vi "DAQ.Create Sample Clock.vi"(8 "error in (no error)":errorcluster, 11 "Instrument.DAQ":refnum<class "Instrument.DAQ.lvclass">) -> (0 "error out":errorcluster, 3 "Instrument.DAQ":refnum<class "Instrument.DAQ.lvclass">)   [LabVIEW 2019, in "Instrument.Lockin.lvlib" / "Instrument.DAQ.lvclass"]
uses:
  Instrument.DAQ.lvclass
  Instrument.DAQ.lvclass/Instrument.DAQ.ctl
  <vilib>/DAQmx/configure/timing.llb/DAQmx Timing (Sample Clock).vi
  <resource>/objmgr/daqmx.rc
panel:
  out "Fs (S/s) 3":dbl[](array[numeric]) format="%#_13g"
  out "Fs (S/s) 2":dbl[](array[numeric]) format="%#_13g"
  out "Output.Onboard Buffer":u32[](array[numeric])
  out "Output.Buffer":u32[](array[numeric])
  out "Input.Onboard Buffer":u32[](array[numeric])
  out "Input.Buffer":u32[](array[numeric])
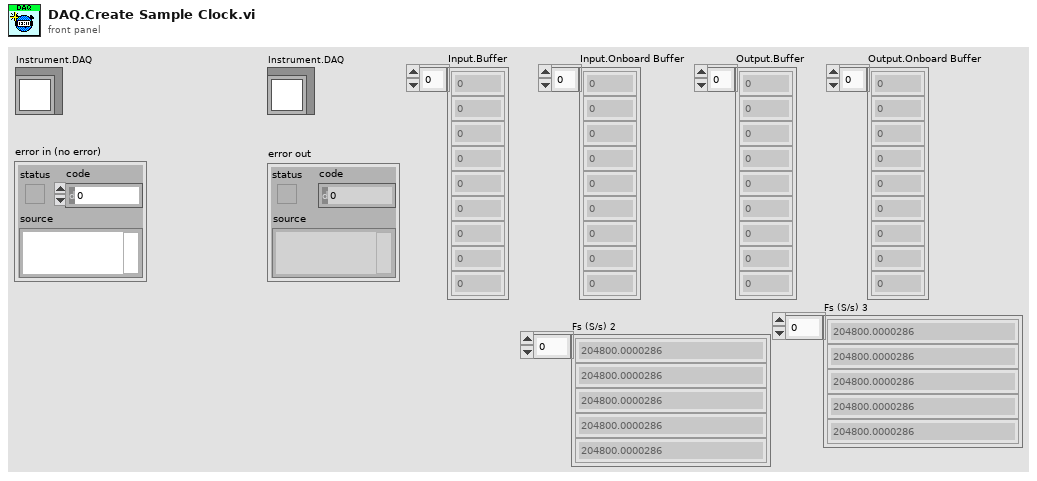
[diagram p1: front panel]
types:
  T1 = typedef "Instrument.Lockin.lvlib/Instrument.DAQ.lvclass/DAQ.Sampling--Cluster.ctl" = cluster{"Sampling":T2, "sample mode":i32, "Fs Mode":T3, "Fs Multiplier":dbl, "Refresh Rate (Hz)":dbl, "Decimation.PreDSP":i32, "Decimation.PostDSP":i32, "Fs.Output":dbl}
  T2 = typedef "Instrument.Lockin.lvlib/Instrument.DAQ.lvclass/DAQ.Sampling.Sampling--Cluster.ctl" = cluster{"Fs":dbl, "#s":i32}
  T3 = typedef "Instrument.Lockin.lvlib/Instrument.DAQ.lvclass/DAQ.Sampling.Fs Mode--enum.ctl" = enum16{"Manual", "Auto Fs", "Max Fs"}
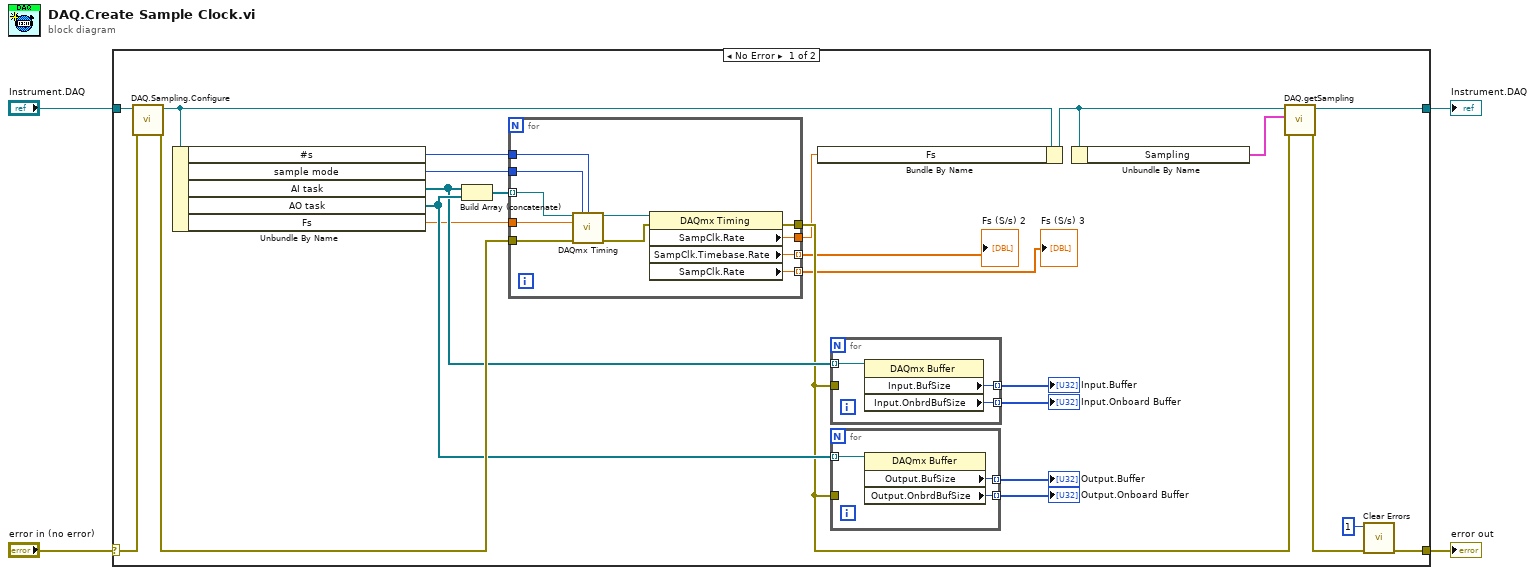
[diagram p0: block diagram]
diagram:
  n1 = case shown="No Error" "error in (no error)" {
    selector: "error in (no error)" -> [w15 w47]
    tunnel: [w7 w47] -> w4
    tunnel: [w14 w46] -> w2
    tunnel: "Instrument.DAQ" -> [w27 w46]
    frame No Error {
      n2 = call "DAQ.Sampling.Configure.vi"("error in (no error)"=w15, "Instrument.DAQ"=w27) -> ("error out"=w25:errorcluster, "Instrument.DAQ out"=w26:refnum<class "Instrument.DAQ.lvclass">)  [unwired: 8 in]
      n3 = Unbundle By Name(w26) -> ("#s"=w16:i32, "sample mode"=w28:i32, "AI task"=w18:refnum<k21>[], "AO task"=w23:refnum<k21>[], "Fs"=w11:dbl)
      n4 = Build Array (concatenate)(w18, w23) -> (w24:refnum<k21>[])
      n5 = for {
        tunnel: w24 -> [w33] mode=indexing
        tunnel: w11 -> [w32]
        tunnel: w25 -> [w31]
        tunnel: [w36] -> w12
        tunnel: [w38] -> w10
        tunnel: w28 -> [w35]
        tunnel: w16 -> [w34]
        tunnel: [w30] -> w9 mode=indexing
        tunnel: [w29] -> w8 mode=indexing
        n6 = call-poly <vilib>:"DAQmx Timing.vi"("task/channels in"=w33, "sample mode"=w35, "samples per channel"=w34, "rate"=w32, "error in"=w31) -> ("task out"=w39:refnum<k21>, "error out"=w37:errorcluster)  [unwired: 9 in]
        n7 = property class="DAQmx Timing"(reference=w39, error in=w37) -> (error out=w36:errorcluster, "SampClk.Rate"=w38:dbl, "SampClk.Timebase.Rate"=w30:dbl, "SampClk.Rate"=w29:dbl)  [unwired: 1 out]
      }
      "Fs (S/s) 2" <- w9
      "Fs (S/s) 3" <- w8
      n8 = Bundle By Name(cluster=w26, "Fs"=w10) -> (w13:refnum<class "Instrument.DAQ.lvclass">)
      n9 = for {
        tunnel: w18 -> [w45] mode=indexing
        tunnel: [w44] -> w22 mode=indexing
        tunnel: [w43] -> w21 mode=indexing
        tunnel: w12 -> [_]
        n10 = property class="DAQmx Buffer"(reference=w45) -> ("Input.BufSize"=w44:u32, "Input.OnbrdBufSize"=w43:u32)  [unwired: 1 in, 2 out]
      }
      "Input.Buffer" <- w22
      "Input.Onboard Buffer" <- w21
      n11 = for {
        tunnel: w23 -> [w42] mode=indexing
        tunnel: [w41] -> w20 mode=indexing
        tunnel: [w40] -> w19 mode=indexing
        tunnel: w12 -> [_]
        n12 = property class="DAQmx Buffer"(reference=w42) -> ("Output.BufSize"=w41:u32, "Output.OnbrdBufSize"=w40:u32)  [unwired: 1 in, 2 out]
      }
      "Output.Buffer" <- w20
      "Output.Onboard Buffer" <- w19
      n13 = Unbundle By Name(w13) -> ("Sampling"=w17:T1)
      n14 = call "DAQ.getSampling.vi"("error in (no error)"=w12, "Sampling"=w17, "Instrument.DAQ"=w13) -> ("error out"=w6:errorcluster, "Instrument.DAQ out"=w14:refnum<class "Instrument.DAQ.lvclass">)  [unwired: 7 in]
      n15 = call <vilib>:"Clear Errors.vi"("error in (no error)"=w6, "specific error code to clear (0: all)"=1) -> ("error out"=w7:errorcluster)  [unwired: 4 in, 1 out]
    }
    frame Error {
    }
  }
  "error out" <- w4
  "Instrument.DAQ" <- w2
